vi "Make Max Stack.vi"(8 "error in (no error)":errorcluster, 10 "Kernel Size":i32, 11 "Image Stack":T1[](array[typedef])) -> (0 "error out":errorcluster, 3 "Max Stack":T1[](array[typedef]))   [LabVIEW 2013]
uses:
  <vilib>/vision/Image Controls.llb/IMAQ Image.ctl
  <vilib>/vision/NI_Vision_Development_Module.lvlib
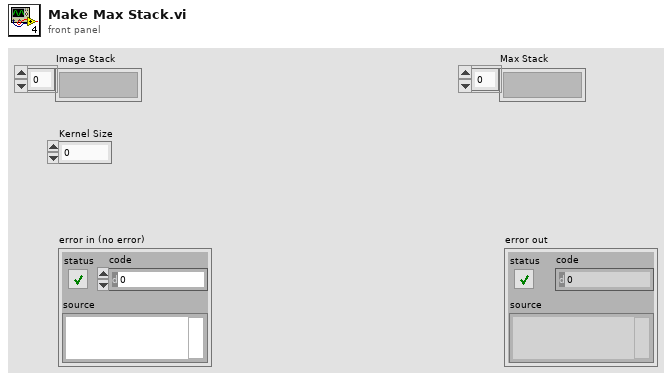
[diagram p1: front panel]
types:
  T1 = typedef "IMAQ Image.ctl" = refnum<image>
  T2 = enum32{"AutoM", "Close", "Dilate", "Erode", "Gradient", "Gradient in", "Gradient out", "HitMiss", "Open", "PClose", "POpen", "Thick", "Thin"}
  T3 = enum32{"Differentiation", "Gradient", "Prewitt", "Roberts", "Sigma", "Sobel"}
  T4 = typedef "Image Type" = u32
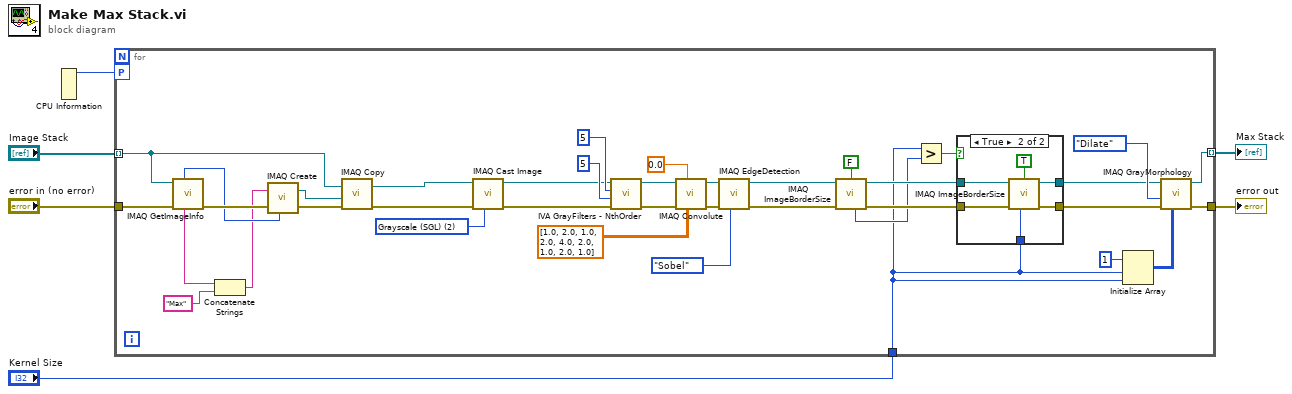
[diagram p0: block diagram]
diagram:
  n1 = CPU Information() -> (4:w1:i32)  [unwired: 3 out]
  n2 = for {
    tunnel: "Image Stack" -> [w38] mode=indexing
    tunnel: [w21] -> w6 mode=indexing
    tunnel: "error in (no error)" -> [w44]
    tunnel: [w20] -> w5
    tunnel: "Kernel Size" -> [w8]
    workers-P: w1 -> [_]
    w29 = T4 2 items=["Grayscale (U8)", "Grayscale (I16)", "Grayscale (SGL)", "Complex (CSG)", "RGB (U32)", "HSL (U32)", "RGB (U64)", "Grayscale (U16)"] ("Image Type")
    n3 = call "IMAQ GetImageInfo"("error in (no error)"=w44, "Image"=w38) -> ("error out"=w43:errorcluster, "Image Name"=w42:string, "Image Type"=w41:T4)  [unwired: 2 in, 5 out]
    n4 = Concatenate Strings(w42, "Max" ("string")) -> (w24:string)
    n5 = call "IMAQ Create"("Image Name"=w24, "Image Type"=w41, "error in (no error)"=w43) -> ("New Image"=w39:T1, "error out"=w40:errorcluster)  [unwired: 2 in]
    n6 = call "IMAQ Copy"("error in (no error)"=w40, "Image Dst"=w39, "Image Src"=w38) -> ("error out"=w27:errorcluster, "Image Dst Out"=w28:T1)  [unwired: 3 in]
    n7 = call "IMAQ Cast Image"("Image Type"=w29, "error in (no error)"=w27, "Image Src"=w28) -> ("error out"=w26:errorcluster, "Image Dst Out"=w25:T1)  [unwired: 3 in, 4 out]
    n8 = call <vilib>:"IVA GrayFilters - NthOrder.vi"("error in"=w26, "Filter size Y"=5, "Filter size X"=5, "Image In"=w25) -> ("error out"=w33:errorcluster, "Image Out"=w34:T1)  [unwired: 6 out]
    n9 = call "IMAQ Convolute"("Kernel"=sgl[][] [[1.0, 2.0, 1.0], [2.0, 4.0, 2.0], [1.0, 2.0, 1.0]], "Divider (kernel sum)"=sgl 0.0 ("Divider"), "error in (no error)"=w33, "Image Src"=w34) -> ("error out"=w30:errorcluster, "Image Dst Out"=w31:T1)  [unwired: 3 in, 3 out]
    n10 = call "IMAQ EdgeDetection"("Method"=T3."Sobel", "error in (no error)"=w30, "Image Src"=w31) -> ("error out"=w11:errorcluster, "Image Dst Out"=w12:T1)  [unwired: 3 in, 4 out]
    n11 = call "IMAQ ImageBorderSize"("Get/Set Status? (Set)"=FALSE, "Image"=w12, "error in (no error)"=w11) -> ("Image Out"=w15:T1, "error out"=w16:errorcluster, "Image border size out"=w14:i32)  [unwired: 1 in]
    n12 = Greater?(x=w8, y=w14) -> (0:w17:bool)
    n13 = case shown="True" w17 {
      tunnel: w16 -> [w45 w51]
      tunnel: w15 -> [w46 w50]
      tunnel: [w46 w49] -> w10
      tunnel: [w45 w48] -> w9
      tunnel: w8 -> [_ w47]
      frame False {
      }
      frame True {
        n14 = call "IMAQ ImageBorderSize"("Get/Set Status? (Set)"=TRUE, "Image"=w50, "Image border size in"=w47, "error in (no error)"=w51) -> ("Image Out"=w49:T1, "error out"=w48:errorcluster)  [unwired: 1 out]
      }
    }
    n15 = Initialize Array(1, w8, w8) -> (w18:i32[][])
    n16 = call "IMAQ GrayMorphology"("Structuring Element"=w18, "error in (no error)"=w9, "Operation"=T2."Dilate", "Image Src"=w10) -> ("error out"=w20:errorcluster, "Image Dst Out"=w21:T1)  [unwired: 6 in]
  }
  "error out" <- w5
  "Max Stack" <- w6
